vi "Pointers_Clear All.vi"(8 "error in (no error)":errorcluster, 11 "(WavBuf) in":refnum<class "(WavBuf).lvclass">) -> (0 "error out":errorcluster, 3 "(WavBuf) out":refnum<class "(WavBuf).lvclass">)   [LabVIEW 2016, in "(WavBuf).lvclass"]
uses:
  (WavBuf).lvclass
  Pointer/((Pointer)).lvclass
  (WavBuf).lvclass/(WavBuf).ctl
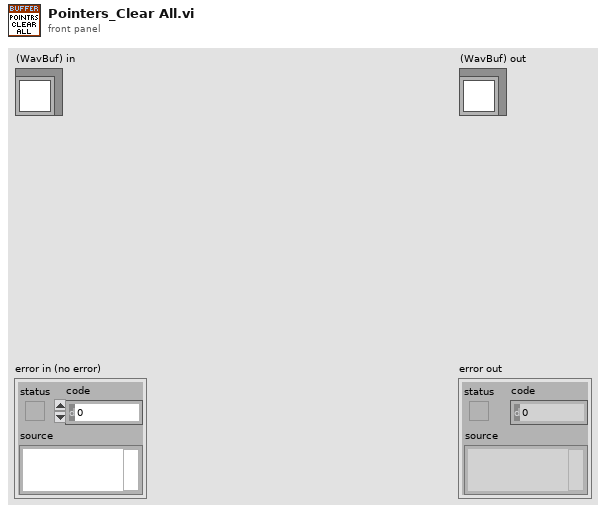
[diagram p1: front panel]
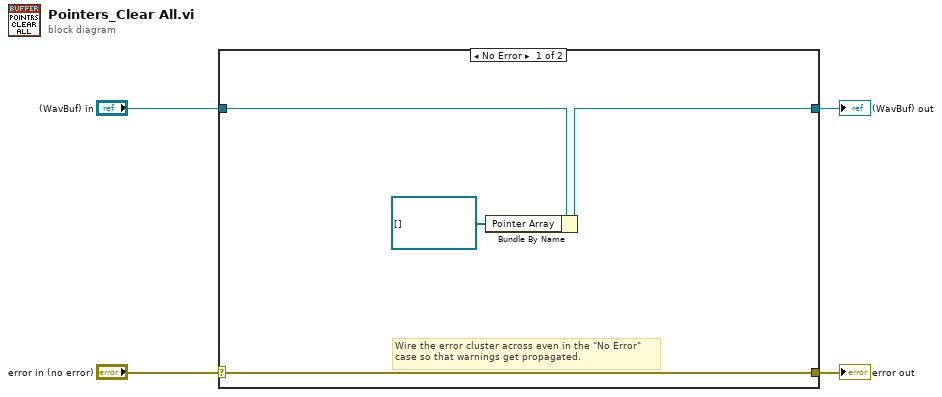
[diagram p0: block diagram]
diagram:
  n1 = case shown="No Error" "error in (no error)" {
    selector: "error in (no error)" -> [w8 w10]
    tunnel: [w8 w10] -> w3
    tunnel: [w6 w9] -> w1
    tunnel: "(WavBuf) in" -> [w7 w9]
    frame No Error {
      # "Wire the error cluster across even in the \"No Error\"\ncase so that warnings get propagated."
      n2 = Bundle By Name(cluster=w7, "Pointer Array"=refnum<class "((Pointer)).lvclass">[] []) -> (w6:refnum<class "(WavBuf).lvclass">)
    }
    frame Error {
    }
  }
  "error out" <- w3
  "(WavBuf) out" <- w1
